vi "Assembler.vi"() -> ()   [LabVIEW 2019]
uses:
  <vilib>/ActorFramework/Message Enqueuer/Message Priority.ctl
  <vilib>/gpm_packages/@cs/mva-viewable/Source/IViewable/IViewable/View Position Enum.ctl
  <vilib>/gpm_packages/@cs/Car-wash/Source/Normal Active Station View/Normal Active Station View/Normal Active Option View.lvclass
  C:/Program Files/National Instruments/LabVIEW 2019/vi.lib/gpm_packages/@cs/Car-wash/Source/Active Station View Definition/Active Station View Definition/Active Option View Definition.lvclass
  <vilib>/gpm_packages/@cs/Car-wash/Source/Car Wash Model/Car Wash Model/Car Wash Model.lvclass
  C:/Program Files/National Instruments/LabVIEW 2019/vi.lib/gpm_packages/@cs/mva-core/Source/IObserver/IObserver/IObserver.lvclass
  C:/Program Files/National Instruments/LabVIEW 2019/vi.lib/gpm_packages/@cs/mva-core/Source/IModel/IModel/IModel.lvclass
  <vilib>/gpm_packages/@cs/Car-wash/Source/Process Model/Process Model.lvclass
  C:/Program Files/National Instruments/LabVIEW 2019/vi.lib/gpm_packages/@cs/Car-wash/Source/iProcess Model/iProcess Model/iProcess Model.lvclass
  <vilib>/gpm_packages/@cs/Car-wash/Source/Simulated Car Position Monitor Model/Simulated Car Position Monitor Model.lvclass
  C:/Program Files/National Instruments/LabVIEW 2019/vi.lib/gpm_packages/@cs/Car-wash/Source/iCar Position Monitor Model/iCar Position Monitor Model/iCar Position Monitor Model.lvclass
  <vilib>/gpm_packages/@cs/Car-wash/Source/Application Types/Option Definition.ctl
  <vilib>/gpm_packages/@cs/Car-wash/Source/Loading View/Loading View.lvclass
  <vilib>/gpm_packages/@cs/Car-wash/Source/Navigation View/Navigation View.lvclass
  <vilib>/gpm_packages/@cs/Car-wash/Source/Process Builder View/Process Builder View.lvclass
  C:/Program Files/National Instruments/LabVIEW 2019/vi.lib/gpm_packages/@cs/Test-executive-builder/Source/Test Executive Builder View/Test Executive Builder View/Test Executive Builder View.lvclass
  <vilib>/gpm_packages/@cs/Car-wash/Source/Process Explorer View/Process Explorer View.lvclass
  C:/Program Files/National Instruments/LabVIEW 2019/vi.lib/gpm_packages/@cs/file-explorer-extension/Source/File Explorer/File Explorer/File Explorer.lvclass
  <vilib>/gpm_packages/@cs/Car-wash/Source/Process Builder Model/Process Builder Model.lvclass
  C:/Program Files/National Instruments/LabVIEW 2019/vi.lib/gpm_packages/@cs/Test-executive-builder/Source/Test Executive Builder Model/Test Executive Builder Model/Test Executive Builder Model.lvclass
  <vilib>/gpm_packages/@cs/Car-wash/Source/Splash Screen Contract Model/Splash Screen Contract Model.lvclass
  C:/Program Files/National Instruments/LabVIEW 2019/vi.lib/gpm_packages/@cs/Car-wash/Source/iSplash Screen Contract Model/iSplash Screen Contract Model.lvclass
  <vilib>/gpm_packages/@cs/Car-wash/Source/Fancy Entry Console View/Fancy Entry Console View/Fancy Entry Console View.lvclass
  C:/Program Files/National Instruments/LabVIEW 2019/vi.lib/gpm_packages/@cs/Car-wash/Source/Entry Console View Definition/Entry Console View Definition/Entry Console View Definition.lvclass
  <vilib>/gpm_packages/@cs/Car-wash/Source/Fancy Car Wash Status View/Fancy Car Wash Status View/Fancy Car Wash Status View.lvclass
  C:/Program Files/National Instruments/LabVIEW 2019/vi.lib/gpm_packages/@cs/Car-wash/Source/Car Wash Status View Definition/Car Wash Status View Definition/Car Wash Status View Definition.lvclass
  <vilib>/gpm_packages/@cs/Car-wash/Source/Fancy Active Option Time Remaining View/Fancy Active Option Elapsed Time View.lvclass
  C:/Program Files/National Instruments/LabVIEW 2019/vi.lib/gpm_packages/@cs/Car-wash/Source/Active Station Time Remaining View Definition/Active Station Time Remaining View Definition/Active Option Elapsed Time View Definition.lvclass
  <vilib>/gpm_packages/@cs/Car-wash/Source/Fancy Car Position Simulation View/Fancy Car Position Simulation View/Fancy Car Position Simulation View.lvclass
  C:/Program Files/National Instruments/LabVIEW 2019/vi.lib/gpm_packages/@cs/Car-wash/Source/Car Position Simulation View Definition/Car Position Simulation View Definition/Car Position Simulation View Definition.lvclass
  <vilib>/gpm_packages/@cs/Car-wash/Source/Fancy Stop Process View/Fancy Stop Process View.lvclass
  C:/Program Files/National Instruments/LabVIEW 2019/vi.lib/gpm_packages/@cs/Car-wash/Source/Stop Process View Definition/Stop Process View Definition.lvclass
  <vilib>/gpm_packages/@cs/persistence/source/XML/XML.lvclass
  C:/Program Files/National Instruments/LabVIEW 2019/vi.lib/gpm_packages/@cs/persistence/source/IPersist/IPersist.lvclass
  <vilib>/gpm_packages/@cs/test-executive/Source/Test Executive/TestExecutive/Test Executive.lvclass
  C:/Program Files/National Instruments/LabVIEW 2019/vi.lib/gpm_packages/@cs/test-executive/Source/Test Executive/ITestExecutive/ITest Executive.lvclass
  <vilib>/gpm_packages/@cs/test-executive/Source/Path Builder/IPath Builder/IPath Builder.lvclass
  <vilib>/gpm_packages/@cs/mva-core/Source/MonitoredMediator/MonitoredMediator/MonitoredMediator.lvclass
  C:/Program Files/National Instruments/LabVIEW 2019/vi.lib/gpm_packages/@cs/mva-core/Source/IMediator/IMediator/IMediator.lvclass
  <vilib>/gpm_packages/@cs/BusMonitor/ListboxBusMonitor/ListboxBusMonitor/ListboxBusMonitor.lvclass/ListboxBusMonitor.ctl
  <vilib>/gpm_packages/@cs/Car-wash/Source/ViewModel/ViewModel/ViewModel.lvclass
  C:/Program Files/National Instruments/LabVIEW 2019/vi.lib/gpm_packages/@cs/mva-viewable/Source/IViewModel/IViewModel/IViewModel.lvclass
  C:/Program Files/National Instruments/LabVIEW 2019/vi.lib/ActorFramework/Actor/Actor.lvclass
  <vilib>/gpm_packages/@cs/mva-core/Source/MonitoredMediator/MonitoredMediator/MonitoredMediator.lvclass/MonitoredMediator.ctl
  <vilib>/gpm_packages/@cs/event-logger/Source/Composed Log/LoggerReference/LoggerReference.lvclass/LoggerReference.ctl
  <vilib>/gpm_packages/@cs/mva-core/Source/IObserver/IObserver/IObserver.lvclass/IObserver.ctl
  <vilib>/gpm_packages/@cs/mva-core/Source/IMediator/IMediator/IMediator.lvclass/IMediator.ctl
  <vilib>/gpm_packages/@cs/mva-viewable/Source/IViewModel/IViewModel/IViewModel.lvclass/IViewModel.ctl
  <vilib>/gpm_packages/@cs/mva-viewable/Source/IViewManager/IViewManager Messages/Launch Nested Views Msg/Launch Nested Views Msg.lvclass/Launch Nested Views Msg.ctl
  <vilib>/gpm_packages/@cs/mva-viewable/Source/IViewManager/IViewManager/IViewManager.lvclass/IViewManager.ctl
  <vilib>/gpm_packages/@cs/mva-viewable/Source/IViewable/IViewable Messages/Open Front Panel Msg/Open Front Panel Msg.lvclass/Open Front Panel Msg.ctl
  <vilib>/ActorFramework/Message Enqueuer/Message Enqueuer.lvclass/Message Enqueuer.ctl
  c5faea81-6703-49a7-b9e4-e5de0ee12b15.vi
  d1888c19-076a-4ff6-8032-cc99172f50c8.vi
  <vilib>/gpm_packages/@cs/mva-core/Source/MonitoredMediator/MonitoredMediator/Private Write BusMonitors.vi
  d1888c19-076a-4ff6-8032-cc99172f50c8.vi/1cb0c31c-b70b-4bde-b060-49cabf9c260e.vi
  <vilib>/gpm_packages/@cs/mva-core/Source/IObserver/IObserver/Configure Observer Logging.vi
  <vilib>/gpm_packages/@cs/mva-viewable/Source/IViewModel/IViewModel/Write Startup Model-View Configuration.vi
  <vilib>/gpm_packages/@cs/mva-core/Source/IMediator/IMediator/Configure Mediator.vi
  <vilib>/ActorFramework/Message Enqueuer/Enqueue.vi
  <vilib>/gpm_packages/@cs/event-logger/Source/Composed Log/LoggerReference/Return Aggregate Queues.vi
  <vilib>/gpm_packages/@cs/event-logger/Source/Composed Log/LoggerReference/Add Aggregate Log.vi
  d1888c19-076a-4ff6-8032-cc99172f50c8.vi/1cb0c31c-b70b-4bde-b060-49cabf9c260e.vi/fb61beb2-99fe-4cb7-b80d-d1e9436b71a7.vi
  <vilib>/gpm_packages/@cs/mva-viewable/Source/IViewManager/IViewManager Messages/Launch Nested Views Msg/Pack Launch Nested Views Msg.vi
  <vilib>/gpm_packages/@cs/mva-viewable/Source/IViewManager/IViewManager/Write Startup Launch Nested Views Msg.vi
  <vilib>/gpm_packages/@cs/event-logger/Source/Composed Log/LoggerReference/Send Add Sink.vi
  <vilib>/gpm_packages/@cs/event-logger/Source/Text File Sink/Text File Sink.lvclass
  C:/Program Files/National Instruments/LabVIEW 2019/vi.lib/gpm_packages/@cs/event-logger/Source/Composed Log/Log Sink/Log Sink.lvclass
  <vilib>/gpm_packages/@cs/Car-wash/Source/Splash Screen ViewManager/Splash Screen ViewManager.lvclass
  C:/Program Files/National Instruments/LabVIEW 2019/vi.lib/gpm_packages/@cs/mva-viewable/Source/IViewable/IViewable/IViewable.lvclass
  <vilib>/gpm_packages/@cs/mva-viewable/Source/IViewModel/IViewModel/IViewModel.lvclass
  C:/Program Files/National Instruments/LabVIEW 2019/vi.lib/gpm_packages/@cs/mva-viewable/Source/IViewManager/IViewManager/IViewManager.lvclass
  <vilib>/gpm_packages/@cs/mva-viewable/Source/IViewable/IViewable Messages/Open Front Panel Msg/Open Front Panel Msg.lvclass
  C:/Program Files/National Instruments/LabVIEW 2019/vi.lib/ActorFramework/Message/Message.lvclass
  <vilib>/gpm_packages/@cs/event-logger/Source/Composed Log/Application Logger/Launch Worker Loop.vi
  <vilib>/gpm_packages/@cs/event-logger/Source/Composed Log/LoggerReference/Initialize Logger Instance.vi
  <vilib>/ActorFramework/Message Priority Queue/Priority Enqueue.vi
  <vilib>/gpm_packages/@cs/BusMonitor/ListboxBusMonitor/ListboxBusMonitor/ListboxBusMonitor.lvclass
  <vilib>/gpm_packages/@cs/event-logger/Source/Composed Log/LoggerReference/LoggerReference.lvclass
  <vilib>/gpm_packages/@cs/event-logger/Source/Composed Log/IErrorFormat/IErrorFormat.lvclass
  <vilib>/gpm_packages/@cs/event-logger/Source/Composed Log/Log Sink/Log Sink.lvclass
  <vilib>/gpm_packages/@cs/mva-viewable/Source/IViewable/IApplicationStyle/IApplicationStyle.lvclass
  <vilib>/gpm_packages/@cs/mva-viewable/Source/IViewManager/IViewManager Messages/Launch Nested Views Msg/Launch Nested Views Msg.lvclass
  <vilib>/ActorFramework/Actor/Actor.lvclass
  <vilib>/ActorFramework/Message Enqueuer/Message Enqueuer.lvclass
  <vilib>/gpm_packages/@cs/mva-viewable/Source/IViewable/IViewable/IViewable.lvclass
  <vilib>/gpm_packages/@cs/Car-wash/Source/Main ViewManager/Main ViewManager/Main ViewManager.lvclass
  <vilib>/gpm_packages/@cs/Car-wash/Source/Car Wash Display ViewManager/Car Wash Display ViewManager/Car Wash Display ViewManager.lvclass
  <vilib>/gpm_packages/@cs/Car-wash/Source/Process Builder ViewManager/Navigation ViewManager.lvclass
  <vilib>/gpm_packages/@cs/Test-executive-builder/Source/Test Executive Builder ViewManager/Test Executive Builder ViewManager/Test Executive Builder ViewManager.lvclass
  <vilib>/gpm_packages/@cs/Test-executive-builder/Source/Test Executive Builder Model/Test Executive Builder Model/Test Executive Builder Model.lvclass
panel:
  out "error out":errorcluster
  in  "Start":bool
  out "Elapsed Time":dbl format="%0.2f"
  in  "stop":bool
  out "Wash Entry":bool
  in  "Wash Options":T1
  in  "Car Position Slider":u8(slide) max=3 scale=0.0..4.0
  out "Car Wash Indicators":T2
  # "Entry Console"
  # "Car Wash Display"
  # "Car Position Simulation"
  # "Pre-Soak\nH-P Wash\nL-P Wax\nSpot Free Rinse"
  # "Underbody Wash\nBug Remover"
  # "Tire Shine\nAir Dry"
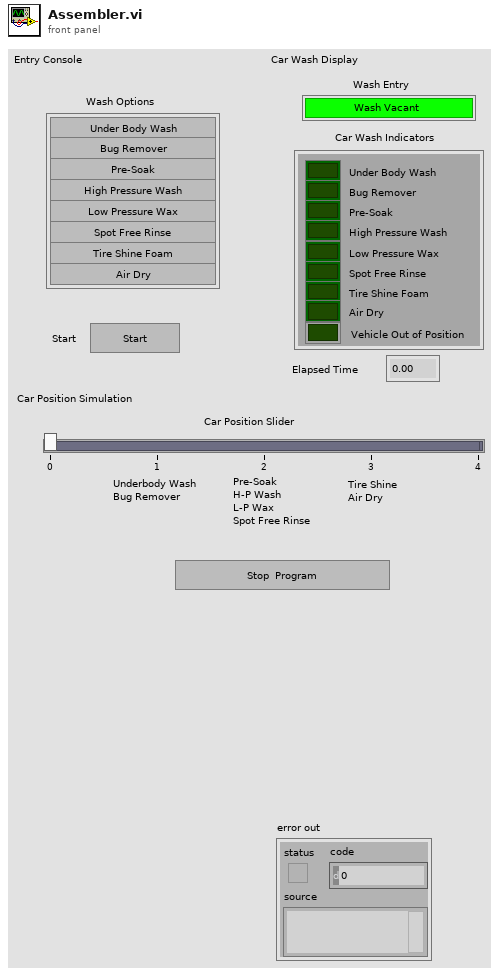
[diagram p1: front panel]
types:
  T1 = cluster{"Underbody Wash":bool, "Bug Remover":bool, "Pre-Soak":bool, "High Pressure Wash":bool, "Low Pressure Wax":bool, "Spot Free Rinse":bool, "Tire Shine Foam":bool, "Air Dry":bool}
  T2 = cluster{"Under Body Wash":bool, "Bug Remover":bool, "Pre-Soak":bool, "High Pressure Wash":bool, "Low Pressure Wax":bool, "Spot Free Rinse":bool, "Tire Shine Foam":bool, "Air Dry":bool, "Vehicle Out of Position":bool}
  T3 = typedef "Option Definition.ctl" = cluster{"Name":string, "Time (mSec)":i32, "Station":u8}
  T4 = typedef "IViewable.lvlib/IViewable.lvclass/View Position Enum.ctl" = enum16{"Centered", "Maximized", "Minimized", "Custom", "Unchanged"}
  T5 = typedef "Actor Framework.lvlib/Message Enqueuer.lvclass/Message Priority.ctl" = enum16{"Low", "Normal", "High"}
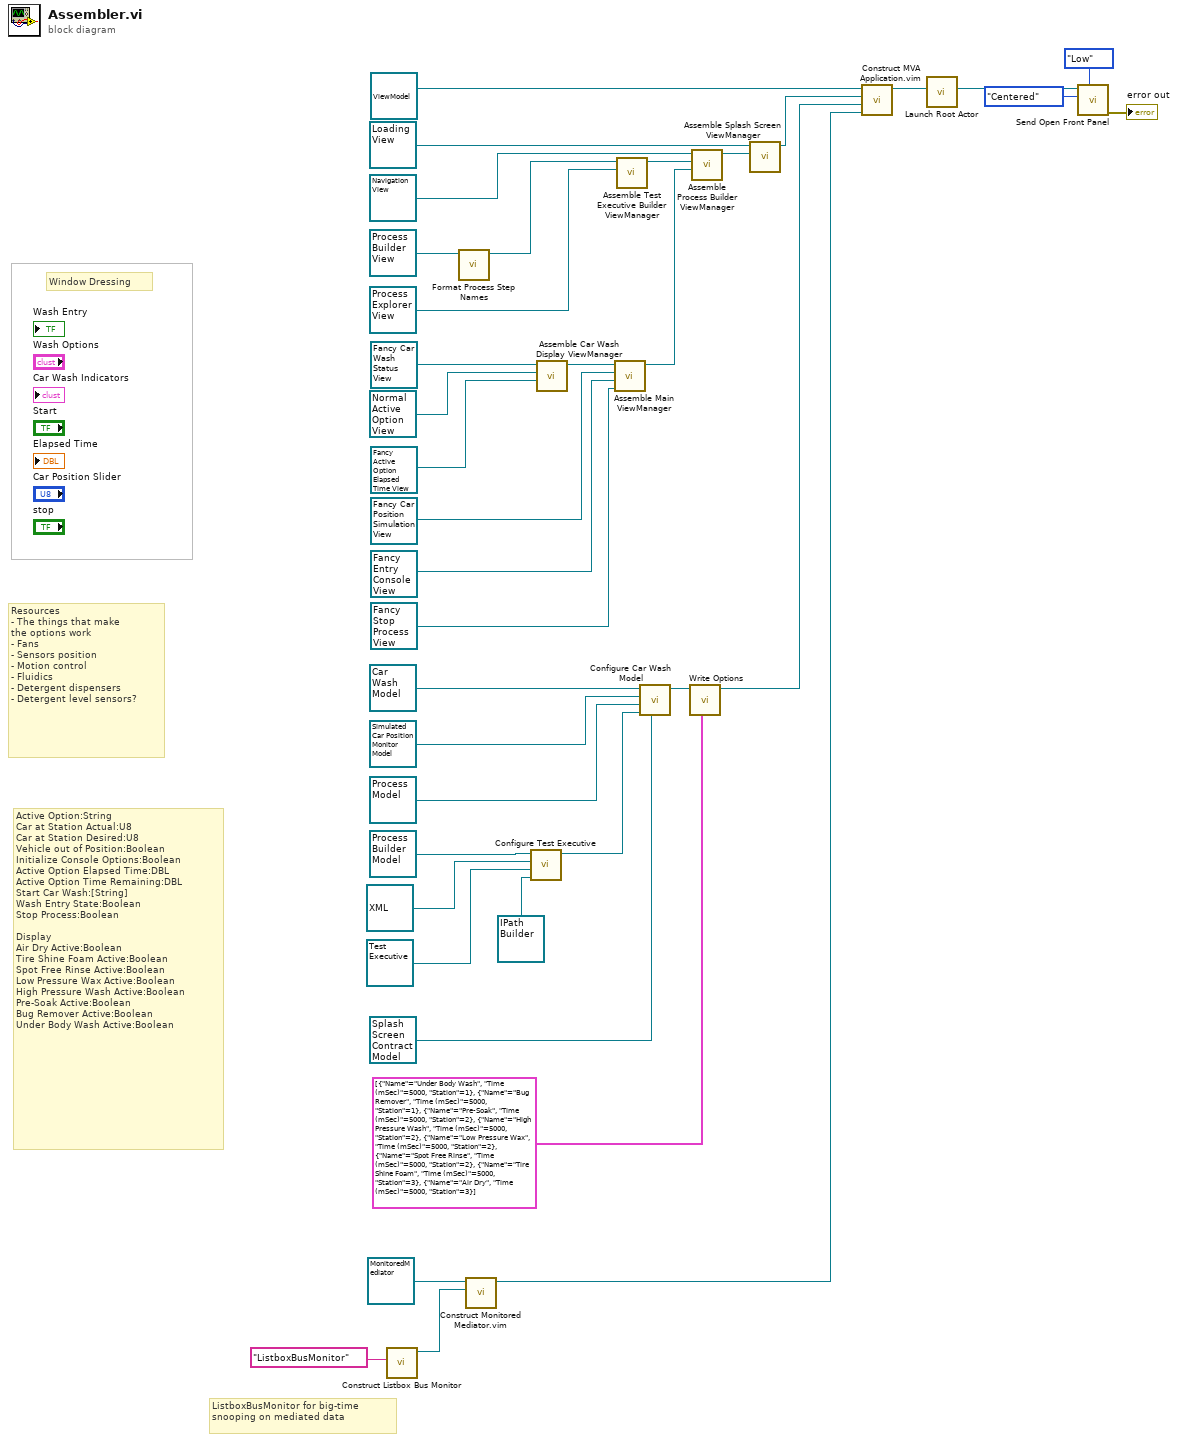
[diagram p0: block diagram]
diagram:
  # "ListboxBusMonitor for big-time\nsnooping on mediated data"
  # "Active Option:String\nCar at Station Actual:U8\nCar at Station Desired:U8\nVehicle out of Position:Boolean\nInitialize Console Options:Boolean\nActive Option Elapsed Time:DBL\nActive Option Time Remaining:DBL\nStart Car Wash:[String]\nWash Entry State:Boolean\nStop Process:Boolean\n\nDisplay\nAir Dry Active:Boolean\nTire Shine Foam Active:Boolean\nSpot Free Rinse Active:Boolean\nLow Pressure Wax Active:Boolean\nHigh Pressure Wash Active:Boolean\nPre-Soak Active:Boolean\nBug Remover Active:Boolean\nUnder Body Wash Active:Boolean"
  # "Resources\n- The things that make\nthe options work\n- Fans\n- Sensors position\n- Motion control\n- Fluidics\n- Detergent dispensers\n- Detergent level sensors?"
  # "Window Dressing"
  n1 = call <vilib>:"Construct Listbox Bus Monitor.vi"("Show Panel Boolean Name"="ListboxBusMonitor") -> ("ListboxBusMonitor out"=w4:refnum<class "ListboxBusMonitor.lvclass">)  [unwired: 10 in]
  n2 = call <vilib>:"Format Process Step Names.vi"("Process Builder View in"=refnum<class "Process Builder View.lvclass"> refnum ("Process Builder View.lvclass")) -> ("Process Builder View out"=w15:refnum<class "Process Builder View.lvclass">)  [unwired: 10 in]
  n3 = call "Construct Monitored Mediator.vim"("Startup Bus Monitor(s)"=w4, "MonitoredMediator in"=refnum<class "MonitoredMediator.lvclass"> refnum ("MonitoredMediator.lvlib:MonitoredMediator.lvclass")) -> ("MonitoredMediator out"=w3:refnum<class "MonitoredMediator.lvclass">)  [unwired: 9 in]
  n4 = call <vilib>:"Configure Test Executive.vi"("Path Builder Type"=refnum<class "IPath Builder.lvclass"> refnum, "Test Executive Type"=refnum<class "Test Executive.lvclass"> refnum ("Test Executive.lvlib:Test Executive.lvclass"), "Persistence Type"=refnum<class "XML.lvclass"> refnum ("XML.lvlib:XML.lvclass"), "Test Executive Builder Model in"=refnum<class "Process Builder Model.lvclass"> refnum ("Process Builder Model.lvclass")) -> ("Test Executive Builder Model out"=w6:refnum<class "Process Builder Model.lvclass">)  [unwired: 7 in]
  n5 = call <vilib>:"Assemble Car Wash Display ViewManager.vi"("Active Station Time Remaining View"=refnum<class "Fancy Active Option Elapsed Time View.lvclass"> refnum ("Fancy Active Option Elapsed Time View.lvclass"), "Active Station View"=refnum<class "Normal Active Option View.lvclass"> refnum ("Normal Active Station View.lvlib:Normal Active Station View.lvclass"), "Car Wash Status View"=refnum<class "Fancy Car Wash Status View.lvclass"> refnum ("Fancy Car Wash Status View.lvclass")) -> ("Car Wash Display ViewManager out"=w33:refnum<class "Car Wash Display ViewManager.lvclass">)  [unwired: 8 in]
  n6 = call <vilib>:"Assemble Main ViewManager.vi"("Stop Process View"=refnum<class "Fancy Stop Process View.lvclass"> refnum ("Fancy Stop Process View.lvclass"), "Entry Console View"=refnum<class "Fancy Entry Console View.lvclass"> refnum ("Fancy Entry Console View.lvclass"), "Car Position Simulation View"=refnum<class "Fancy Car Position Simulation View.lvclass"> refnum ("Fancy Car Position Simulation View.lvclass"), "Car Wash Display ViewManager"=w33) -> ("Main ViewManager out"=w20:refnum<class "Main ViewManager.lvclass">)  [unwired: 7 in]
  n7 = call <vilib>:"Assemble Test Executive Builder ViewManager.vi"("File Explorer View"=refnum<class "Process Explorer View.lvclass"> refnum ("Process Explorer View.lvclass"), "Test Executive Builder View"=w15) -> ("Test Executive Builder ViewManager out"=w7:refnum<class "Test Executive Builder ViewManager.lvclass">)  [unwired: 9 in]
  n8 = call <vilib>:"Configure Car Wash Model.vi"("Splash Screen Contract Model Type"=refnum<class "Splash Screen Contract Model.lvclass"> refnum ("Splash Screen Contract Model.lvclass"), "Process Builder Type"=w6, "Process Model Type"=refnum<class "Process Model.lvclass"> refnum ("Process Model.lvclass"), "Car Position Monitor Type"=refnum<class "Simulated Car Position Monitor Model.lvclass"> refnum ("Car Position Monitor Model.lvclass"), "Car Wash Model in"=refnum<class "Car Wash Model.lvclass"> refnum ("Car Wash Model.lvlib:Car Wash Model.lvclass")) -> ("Car Wash Model out"=w28:refnum<class "Car Wash Model.lvclass">)  [unwired: 6 in]
  n9 = call <vilib>:"Write Options.vi"("Options"=T3[] [{"Name"="Under Body Wash", "Time (mSec)"=5000, "Station"=1}, {"Name"="Bug Remover", "Time (mSec)"=5000, "Station"=1}, {"Name"="Pre-Soak", "Time (mSec)"=5000, "Station"=2}, {"Name"="High Pressure Wash", "Time (mSec)"=5000, "Station"=2}, {"Name"="Low Pressure Wax", "Time (mSec)"=5000, "Station"=2}, {"Name"="Spot Free Rinse", "Time (mSec)"=5000, "Station"=2}, {"Name"="Tire Shine Foam", "Time (mSec)"=5000, "Station"=3}, {"Name"="Air Dry", "Time (mSec)"=5000, "Station"=3}], "Car Wash Model in"=w28) -> ("Car Wash Model out"=w27:refnum<class "Car Wash Model.lvclass">)  [unwired: 9 in]
  n10 = call <vilib>:"Assemble Process Builder ViewManager.vi"("Main ViewManager"=w20, "Process Builder ViewManager"=w7, "Navigation View.lvclass"=refnum<class "Navigation View.lvclass"> refnum) -> ("Main ViewManager out"=w24:refnum<class "Navigation ViewManager.lvclass">)  [unwired: 8 in]
  n11 = call <vilib>:"Assemble Splash Screen ViewManager.vi"("Process Builder ViewManager"=w24, "Loading View"=refnum<class "Loading View.lvclass"> refnum ("Loading View.lvclass")) -> ("Splash Screen ViewManager out"=w8:refnum<class "Splash Screen ViewManager.lvclass">)  [unwired: 9 in]
  n12 = call "Construct MVA Application.vim"("Mediator Type"=w3, "Model Type"=w27, "Startup View Configuration"=w8, "IViewModel In"=refnum<class "ViewModel.lvclass"> refnum ("ViewModel.lvclass")) -> ("IViewModel Out"=w38:refnum<class "ViewModel.lvclass">)  [unwired: 7 in]
  n13 = call <vilib>:"Launch Root Actor.vi"("Actor"=w38) -> ("Actor's Enqueuer"=w37:refnum<class "Message Enqueuer.lvclass">)  [unwired: 9 in, 1 out]
  n14 = call <vilib>:"Send Open Front Panel.vi"("Message Priority (Normal)"=Message_Priority."Low", "Position"=View_Position_Enum."Centered", "Message Enqueuer"=w37) -> ("error out"=→"error out":errorcluster)  [unwired: 7 in, 1 out]
